vi "DAC Stop.vi"(8 "error in (no error)":errorcluster, 11 "DAC Keller Diff P 23X in":refnum<class "DAC Keller Diff P 23X.lvclass">) -> (0 "error out":errorcluster, 3 "DAC Keller Diff P 23X out":refnum<class "DAC Keller Diff P 23X.lvclass">)   [LabVIEW 2019, in "DAC.lvlib" / "DAC Keller Diff P 23X.lvclass"]
uses:
  DAC Keller Diff P 23X.lvclass
  C:/Users/wg/Documents/LV_Projects/test-stand/App/DAC/DAC.lvclass
  DAC.lvclass/DAC.ctl
  DAC Keller Diff P 23X.lvclass/DAC Keller Diff P 23X.ctl
  DAC.lvclass
  <instrlib>/_KELLER RS485 Library/KELLER RS485 Library.lvlib
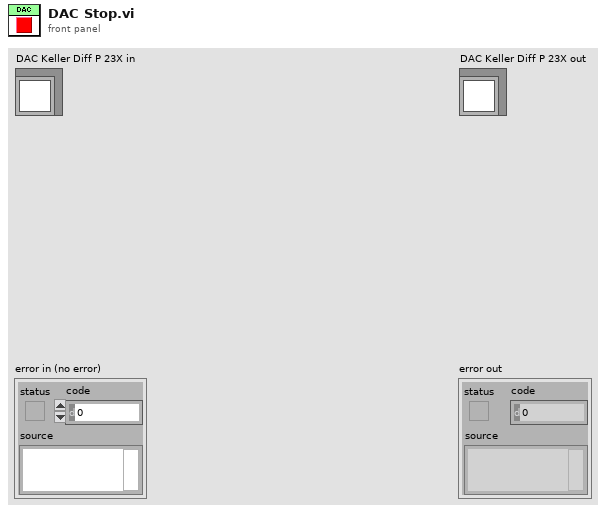
[diagram p1: front panel]
types:
  T1 = typedef "KELLER RS485 Library.lvlib/Bus.ctl" = cluster{"VISA":refnum<visa-resource-name>, "Baud Rate ":T2, "Timeout":u32, "Echo?":bool, "Wait before transmit":u32}
  T2 = typedef "KELLER RS485 Library.lvlib/Baud Rate.ctl" = enum16{"9600bd", "115200bd"}
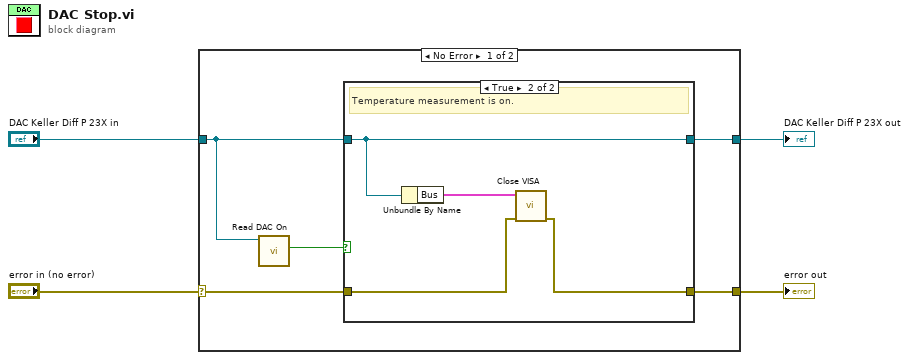
[diagram p0: block diagram]
diagram:
  n1 = case shown="No Error" "error in (no error)" {
    selector: "error in (no error)" -> [w6 w17]
    tunnel: [w5 w17] -> w1
    tunnel: [w7 w16] -> w3
    tunnel: "DAC Keller Diff P 23X in" -> [w9 w16]
    frame No Error {
      n2 = call "Read DAC On.vi"("DAC in"=w9) -> ("DAC On"=w8:bool)  [unwired: 8 in, 2 out]
      n3 = case shown="True" w8 {
        tunnel: w9 -> [w11 w15]
        tunnel: [w11 w15] -> w7
        tunnel: w6 -> [w10 w12]
        tunnel: [w10 w13] -> w5
        frame False {
          # "Temperature measurement is off."
        }
        frame True {
          # "Temperature measurement is on."
          n4 = Unbundle By Name(w15) -> ("Bus"=w14:T1)
          n5 = call <instrlib>:"Close VISA.vi"("error in (no error)"=w12, "Bus in"=w14) -> ("error out"=w13:errorcluster)  [unwired: 9 in]
        }
      }
    }
    frame Error {
    }
  }
  "error out" <- w1
  "DAC Keller Diff P 23X out" <- w3
